vi "NN_Get_Datasets_Path.vi"() -> (3 "Datasets path":path)   [LabVIEW 2020]
doc: "Example helper VI.\nReturns path to pretrained NN models examples."
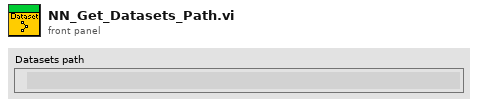
[diagram p1: front panel]
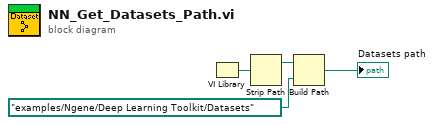
[diagram p0: block diagram]
diagram:
  n1 = VI Library() -> (path=w4:path)
  n2 = Strip Path(path=w4) -> (stripped path=w3:path)  [unwired: 1 out]
  n3 = Build Path(base path=w3, name or relative path=path "examples/Ngene/Deep Learning Toolkit/Datasets" ("stripped path")) -> (appended path=→"Datasets path":path)
